vi "Get Temp Sensor Type.vi"(8 "error in (no error)":errorcluster, 11 "VISA resource name":refnum<visa-resource-name>) -> (0 "error out":errorcluster, 2 "Temp Sensor Type":i32, 3 "VISA resource name out":refnum<visa-resource-name>)   [LabVIEW 2014, in "Fluke 5XXX Series Multicalibrators.lvlib"]
doc: "This VI returns the temperature sensor type thermocouple (TC) or Resistance Temperature Detector (RTD) for temperature measurements.\n\nNote:\n\nThis VI is available only for instrument models 5500A and 5520A."
uses:
  Fluke 5XXX Series Multicalibrators.lvlib
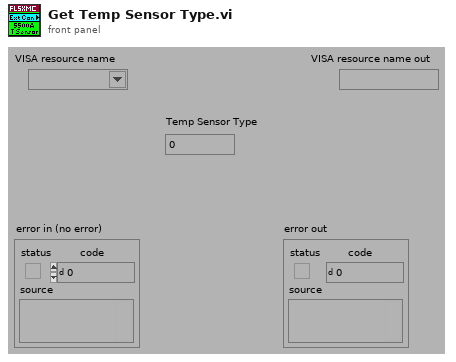
[diagram p1: front panel]
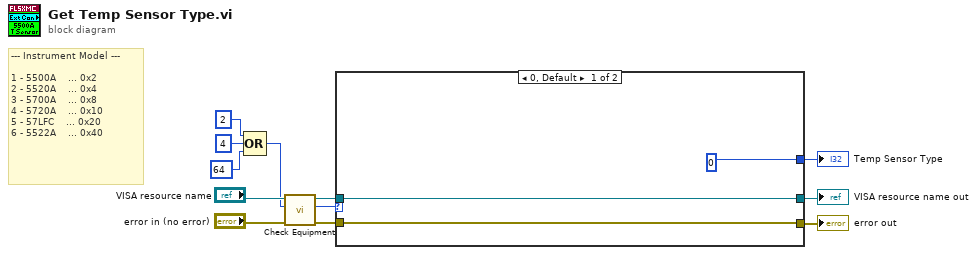
[diagram p0: block diagram]
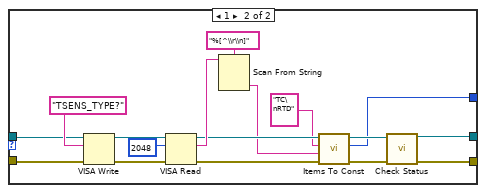
[diagram p2: hidden frame]
diagram:
  # "--- Instrument Model ---\n\n1 - 5500A    ... 0x2\n2 - 5520A    ... 0x4\n3 - 5700A    ... 0x8\n4 - 5720A    ... 0x10\n5 - 57LFC    ... 0x20\n6 - 5522A    ... 0x40"
  n1 = Compound Arithmetic op=OR(2 ("Numeric"), 4 ("Numeric"), 64 ("Numeric")) -> (w1:i32)
  n2 = call "Check Equipment.vi"("error in (no error)"="error in (no error)", "Bit Mask"=w1, "VISA resource name"="VISA resource name") -> ("error out"=w12:errorcluster, "Present?"=w11:u32, "VISA resource name out"=w10:refnum<visa-resource-name>)  [unwired: 6 in]
  n3 = case shown="0, Default" w11 {
    tunnel: [w15 w26] -> w7
    tunnel: [w14 w25] -> w6
    tunnel: w12 -> [w15 w28]
    tunnel: w10 -> [w14 w27]
    tunnel: [u16 0 w16] -> w5
    frame 0, Default {
    }
    frame 1 {
      n4 = VISA Write(VISA resource name=w27, write buffer="TSENS_TYPE?", error in (no error)=w28) -> (VISA resource name out=w31:refnum<visa-resource-name>, error out=w30:errorcluster)  [unwired: 1 out]
      n5 = VISA Read(VISA resource name=w31, byte count=u32 2048 ("byte count (0)"), error in (no error)=w30) -> (VISA resource name out=w20:refnum<visa-resource-name>, read buffer=w23:string, error out=w21:errorcluster)  [unwired: 1 out]
      n6 = Scan From String(format string="%[^\\r\\n]", input string=w23) -> (output 1=w18:string)  [unwired: 3 in, 3 out]
      n7 = call "Items To Const.vi"("error in (no error)"=w21, "String Item"=w18, "Multi-Line String"="TC\nRTD", "VISA resource name"=w20) -> ("error out"=w22:errorcluster, "Index"=w16:i32, "VISA resource name out"=w19:refnum<visa-resource-name>)  [unwired: 5 in]
      n8 = call "Check Status.vi"("VISA resource name"=w19, "error in (no error)"=w22) -> ("VISA resource name out"=w25:refnum<visa-resource-name>, "error out"=w26:errorcluster)  [unwired: 12 in]
    }
  }
  "Temp Sensor Type" <- w5
  "VISA resource name out" <- w6
  "error out" <- w7
